vi "Open Playback Files Crop Utility.vi"(8 "error in (no error)":errorcluster, 11 "Frame Grabber Data In":T2={"Camera Session"="", "Frame"=refnum, "AVI Refnum"=refnum, "Codecs"=[], "Frame number"=0, "Tracking File Refnum"=refnum, "Tick Count"=0, "Probe Object"=refnum, "Playback Probe Data"=[], "Rigid Body"={"Position"={"x (mm)"=0.0, "y (mm)"=0.0, "z (mm)"=0.0}, "Orientation"={"Pitch (rad)"=0.0, "Yaw (rad)"=0.0, "Roll (rad)"=0.0}, "Quaternion"={"qx"=0.0, "qy"=0.0, "qz"=0.0, "qw"=0.0}, "Tracked?"=FALSE}, "Total no frames playback"=0, "Video FPS"=0.0, "Camera connected?"=FALSE, "Scene"=refnum, "Cropped Frame"=refnum, "Tracker FPS"=0.0, "Crop ROI"=[], "Presentation Values"=[], "Elapsed time (ms)"=0, "Camera frames playback"=0, "Refnums"={"Live Refnum"=refnum, "Record Refnum"=refnum, "Playback Refnum"=refnum, "Frame Slider Refnum"=refnum, "Pause Refnum"=refnum, "Home Refnum"=refnum, "Set Crop Refnum"=refnum, "Clear Crop Refnum"=refnum, "stop refnum"=refnum, "Playback Rate Refnum"=refnum, "Presentation Refnum"=refnum, "Crop Time Frame Slider Refnum"=refnum, "Cancel Save Refnum"=refnum, "Reverse Playback Refnum"=refnum, "Recording Settings Refnum"=refnum, "Continuous Playback Refnum"=refnum, "Annotation Refnum"=refnum, "Export All Refnum"=refnum, "Export List Refnum"=refnum, "Fill List Refnum"=refnum, "Save Crop Refnum"=refnum, "Skip Forward Refnum"=refnum, "Skip Backward Refnum"=refnum, "Single Annotation Refnum"=refnum, "Load Video Refnum"=refnum, "Set Start Refnum"=refnum, "Set End Refnum"=refnum, "Add to List Refnum"=refnum, "List of Annotations Refnum"=refnum, "Camera Frame Refnum"=refnum, "Load Image Refnum"=refnum, "Saving Refnum"=refnum}, "Dimensions"={"Probe Dimensions"={"Probe Width"=0.0, "Probe Depth"=1.0, "Probe Height"=0.0}, "Room Dimensions"={"Room Width"=0.0, "Room Depth"=0.0, "Room Height"=0.0}}, "Playback Data As Strings"=[], "Cropped Tracking File Refnum"=refnum, "Cropped AVI Refnum"=refnum, "Header"=[], "Total euclidian distance"=0.0, "Annotation File Path"=path "", "Playback File Path"=path "", "Size per frame"=0.0, "Ground Truth File Refnum"=refnum, "Annotation Array"=[], "Annotation TIFFs Folder"=path "", "overwriting open file?"=FALSE, "Image Sequence"=[], "Video/Image Flag"=enum."Playback Video Frame", "Image sequence?"=FALSE, "Image sequence filenames"=[], "Mask"=refnum}) -> (0 "error out":errorcluster, 1 "Playback Video":path, 2 "both exist and open?":bool, 3 "Frame Grabber Data Out":T2={"Camera Session"="", "Frame"=refnum, "AVI Refnum"=refnum, "Codecs"=[], "Frame number"=0, "Tracking File Refnum"=refnum, "Tick Count"=0, "Probe Object"=refnum, "Playback Probe Data"=[], "Rigid Body"={"Position"={"x (mm)"=0.0, "y (mm)"=0.0, "z (mm)"=0.0}, "Orientation"={"Pitch (rad)"=0.0, "Yaw (rad)"=0.0, "Roll (rad)"=0.0}, "Quaternion"={"qx"=0.0, "qy"=0.0, "qz"=0.0, "qw"=0.0}, "Tracked?"=FALSE}, "Total no frames playback"=0, "Video FPS"=0.0, "Camera connected?"=FALSE, "Scene"=refnum, "Cropped Frame"=refnum, "Tracker FPS"=0.0, "Crop ROI"=[], "Presentation Values"=[], "Elapsed time (ms)"=0, "Camera frames playback"=0, "Refnums"={"Live Refnum"=refnum, "Record Refnum"=refnum, "Playback Refnum"=refnum, "Frame Slider Refnum"=refnum, "Pause Refnum"=refnum, "Home Refnum"=refnum, "Set Crop Refnum"=refnum, "Clear Crop Refnum"=refnum, "stop refnum"=refnum, "Playback Rate Refnum"=refnum, "Presentation Refnum"=refnum, "Crop Time Frame Slider Refnum"=refnum, "Cancel Save Refnum"=refnum, "Reverse Playback Refnum"=refnum, "Recording Settings Refnum"=refnum, "Continuous Playback Refnum"=refnum, "Annotation Refnum"=refnum, "Export All Refnum"=refnum, "Export List Refnum"=refnum, "Fill List Refnum"=refnum, "Save Crop Refnum"=refnum, "Skip Forward Refnum"=refnum, "Skip Backward Refnum"=refnum, "Single Annotation Refnum"=refnum, "Load Video Refnum"=refnum, "Set Start Refnum"=refnum, "Set End Refnum"=refnum, "Add to List Refnum"=refnum, "List of Annotations Refnum"=refnum, "Camera Frame Refnum"=refnum, "Load Image Refnum"=refnum, "Saving Refnum"=refnum}, "Dimensions"={"Probe Dimensions"={"Probe Width"=0.0, "Probe Depth"=1.0, "Probe Height"=0.0}, "Room Dimensions"={"Room Width"=0.0, "Room Depth"=0.0, "Room Height"=0.0}}, "Playback Data As Strings"=[], "Cropped Tracking File Refnum"=refnum, "Cropped AVI Refnum"=refnum, "Header"=[], "Total euclidian distance"=0.0, "Annotation File Path"=path "", "Playback File Path"=path "", "Size per frame"=0.0, "Ground Truth File Refnum"=refnum, "Annotation Array"=[], "Annotation TIFFs Folder"=path "", "overwriting open file?"=FALSE, "Image Sequence"=[], "Video/Image Flag"=enum."Playback Video Frame", "Image sequence?"=FALSE, "Image sequence filenames"=[], "Mask"=refnum}, 4 "Annotation List":T1[](array[typedef]) {"Frame Start" min=0}, 5 "Number of Playback Frames":i32, 7 "Number of Camera Frames":u32)   [LabVIEW 2017]
uses:
  Controls/Frame Grabber Data.ctl
  <vilib>/userdefined/High Color/IMAQdx.ctl
  <vilib>/vision/Image Controls.llb/IMAQ Image.ctl
  <vilib>/vision/Avi.llb/IMAQ AVI2 Refnum.ctl
  Controls/Rigid Body Info.ctl
  Controls/Position.ctl
  Controls/Orientation.ctl
  Controls/Refnums.ctl
  Controls/Recording Settings.ctl
  Controls/Operator Settings.ctl
  Controls/Operator.ctl
  Controls/Patient Settings.ctl
  Controls/Dimensions.ctl
  Controls/Room Dimensions.ctl
  Controls/Crop Video State.ctl
  Controls/Annotation Sequence Details.ctl
  <vilib>/Utility/file.llb/Read Delimited Spreadsheet (string).vi
  <vilib>/vision/NI_Vision_Development_Module.lvlib
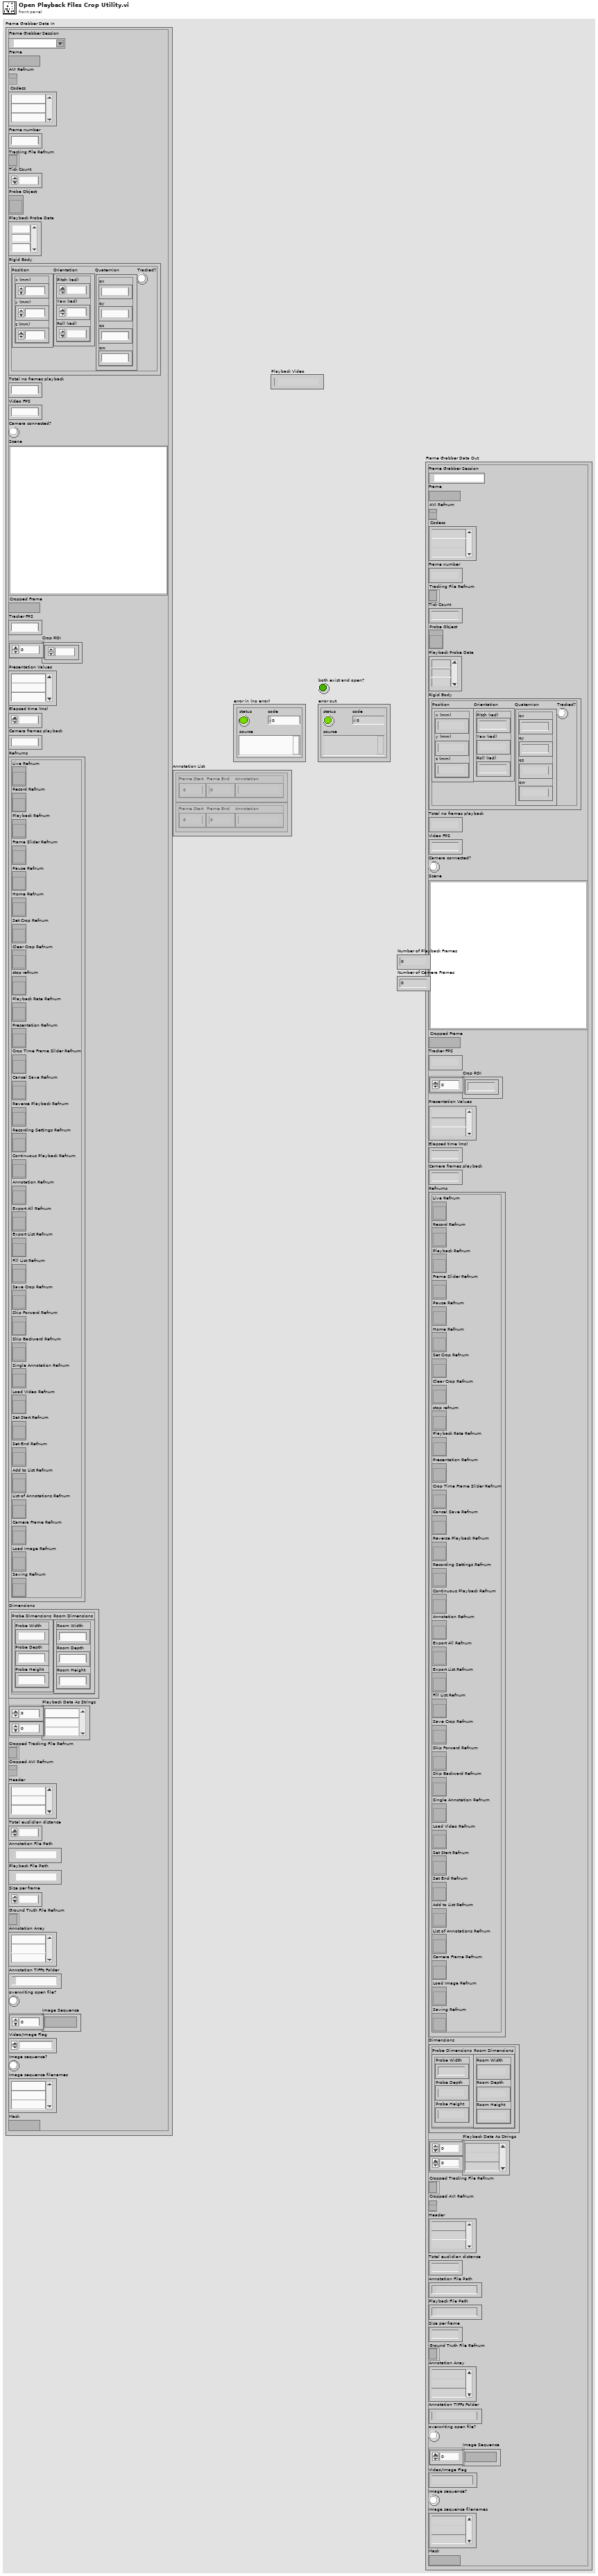
[diagram p1: front panel]
types:
  T1 = typedef "Annotation Sequence Details.ctl" = cluster{"Frame Start":i32, "Frame End":i32, "Annotation":string}
  T2 = typedef "Frame Grabber Data.ctl" = cluster{"Camera Session":T3, "Frame":T4, "AVI Refnum":T5, "Codecs":string[], "Frame number":u32, "Tracking File Refnum":refnum<file>, "Tick Count":u32, "Probe Object":refnum<vi>, "Playback Probe Data":dbl[][], "Rigid Body":T6, "Total no frames playback":i32, "Video FPS":dbl, "Camera connected?":bool, "Scene":refnum<vi>, "Cropped Frame":T4, "Tracker FPS":dbl, "Crop ROI":i32[], "Presentation Values":string[], "Elapsed time (ms)":u32, "Camera frames playback":u32, "Refnums":T9, "Dimensions":T10, "Playback Data As Strings":string[][], "Cropped Tracking File Refnum":refnum<file>, "Cropped AVI Refnum":T5, "Header":string[], "Total euclidian distance":dbl, "Annotation File Path":path, "Playback File Path":path, "Size per frame":dbl, "Ground Truth File Refnum":refnum<file>, "Annotation Array":string[], "Annotation TIFFs Folder":path, "overwriting open file?":bool, "Image Sequence":T4[], "Video/Image Flag":T12, "Image sequence?":bool, "Image sequence filenames":string[], "Mask":T4}
  T3 = typedef "IMAQdx.ctl" = refnum<k21>
  T4 = typedef "IMAQ Image.ctl" = refnum<image>
  T5 = typedef "IMAQ AVI2 Refnum.ctl" = refnum<k20>
  T6 = typedef "Rigid Body Info.ctl" = cluster{"Position":T7, "Orientation":T8, "Quaternion":cluster{"qx":sgl, "qy":sgl, "qz":sgl, "qw":sgl}, "Tracked?":bool}
  T7 = typedef "Position.ctl" = cluster{"x (mm)":sgl, "y (mm)":sgl, "z (mm)":sgl}
  T8 = typedef "Orientation.ctl" = cluster{"Pitch (rad)":sgl, "Yaw (rad)":sgl, "Roll (rad)":sgl}
  T9 = typedef "Refnums.ctl" = cluster{"Live Refnum":refnum<vi>, "Record Refnum":refnum<vi>, "Playback Refnum":refnum<vi>, "Frame Slider Refnum":refnum<vi>, "Pause Refnum":refnum<vi>, "Home Refnum":refnum<vi>, "Set Crop Refnum":refnum<vi>, "Clear Crop Refnum":refnum<vi>, "stop refnum":refnum<vi>, "Playback Rate Refnum":refnum<vi>, "Presentation Refnum":refnum<vi>, "Crop Time Frame Slider Refnum":refnum<vi>, "Cancel Save Refnum":refnum<vi>, "Reverse Playback Refnum":refnum<vi>, "Recording Settings Refnum":refnum<vi>, "Continuous Playback Refnum":refnum<vi>, "Annotation Refnum":refnum<vi>, "Export All Refnum":refnum<vi>, "Export List Refnum":refnum<vi>, "Fill List Refnum":refnum<vi>, "Save Crop Refnum":refnum<vi>, "Skip Forward Refnum":refnum<vi>, "Skip Backward Refnum":refnum<vi>, "Single Annotation Refnum":refnum<vi>, "Load Video Refnum":refnum<vi>, "Set Start Refnum":refnum<vi>, "Set End Refnum":refnum<vi>, "Add to List Refnum":refnum<vi>, "List of Annotations Refnum":refnum<vi>, "Camera Frame Refnum":refnum<vi>, "Load Image Refnum":refnum<vi>, "Saving Refnum":refnum<vi>}
  T10 = typedef "Dimensions.ctl" = cluster{"Probe Dimensions":cluster{"Probe Width":sgl, "Probe Depth":sgl, "Probe Height":sgl}, "Room Dimensions":T11}
  T11 = typedef "Room Dimensions.ctl" = cluster{"Room Width":dbl, "Room Depth":dbl, "Room Height":dbl}
  T12 = typedef "Crop Video State.ctl" = enum16{"Init", "Wait", "Load Image", "Load Video", "Play/Pause", "Playback Video Frame", "Display Image", "Save Image Sequence", "Save Video", "Export List", "Export All", "Close", "Set Crop Area", "Reset Crop Area", "Crop Inside", "Crop Outside", "Multi-Crop", "Re-Open Files", "Annotate Frame", "Annotate Clip", "Add to List", "Fill List", "Set Start", "Set End", "Error Handling", "Shutdown"}
  T13 = enum16{"open", "replace", "create", "open or create", "replace or create", "replace or create with confirmation"}
  T14 = typedef "IMAQ Rectangle" = cluster{"Left":i32, "Top":i32, "Right":i32, "Bottom":i32, "Rotation":dbl}
  T15 = enum8{"Enabled", "Disabled", "Disabled and Grayed Out"}
  T16 = cluster{"Width":u32, "Height":u32, "Frames Per Second":u32, "Codec":string, "Has Data":bool}
  T17 = cluster{"Scale.Range:Minimum":i32, "Number of Frames":u32, "Scale.Range:Minimum":i32}
  T18 = typedef "ROI Descriptor" = cluster{"Global Rectangle":i32[], "Contours":cluster{"ID":enum32{"External", "Internal"}, "Type":u32, "Coordinates":i32[]}[]}
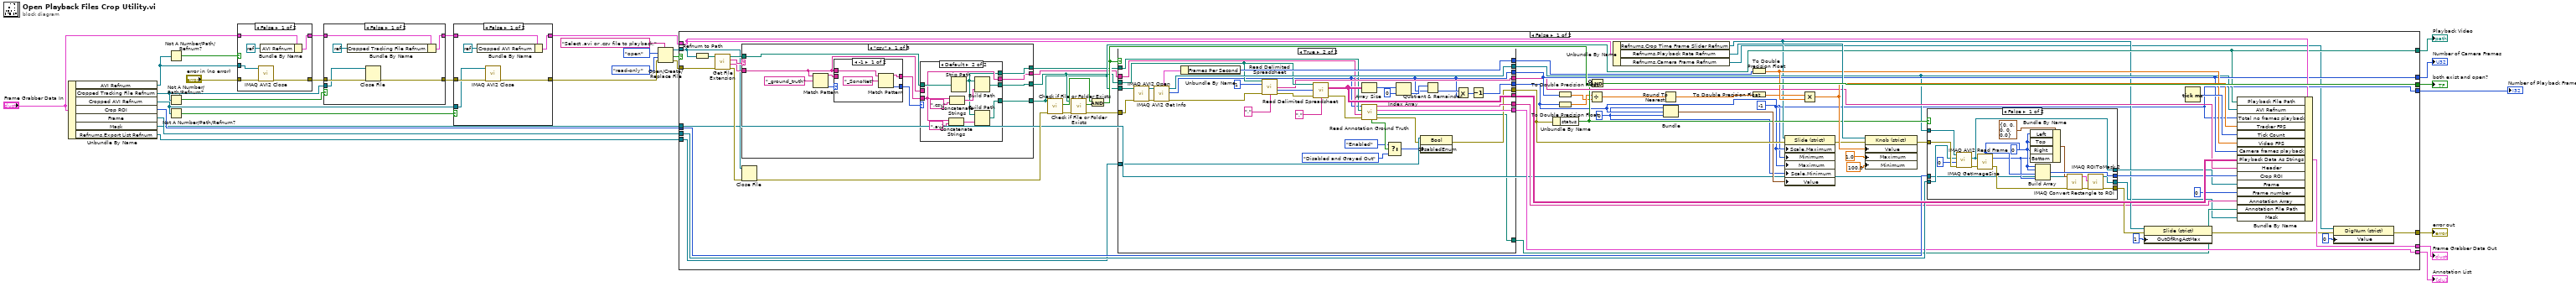
[diagram p0: block diagram]
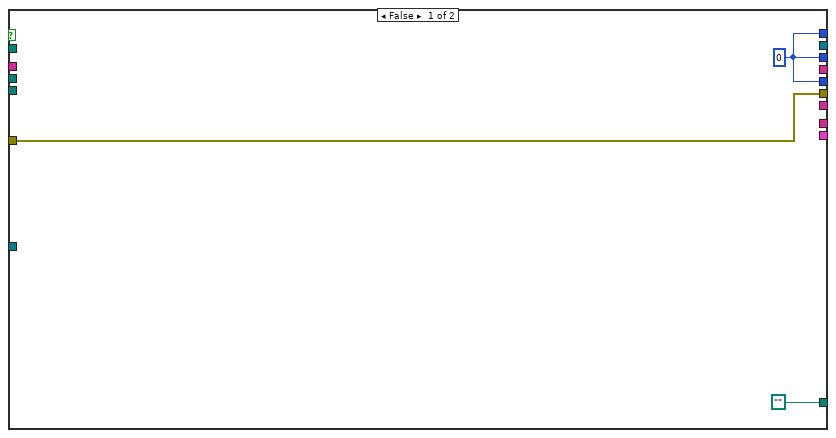
[diagram p6: hidden frame]
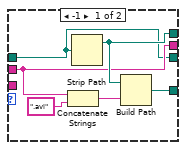
[diagram p8: hidden frame]
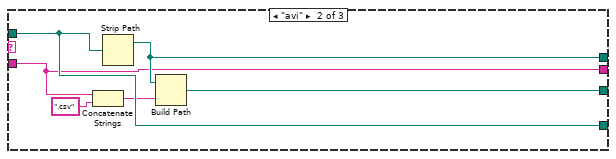
[diagram p9: hidden frame]
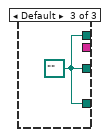
[diagram p10: hidden frame]
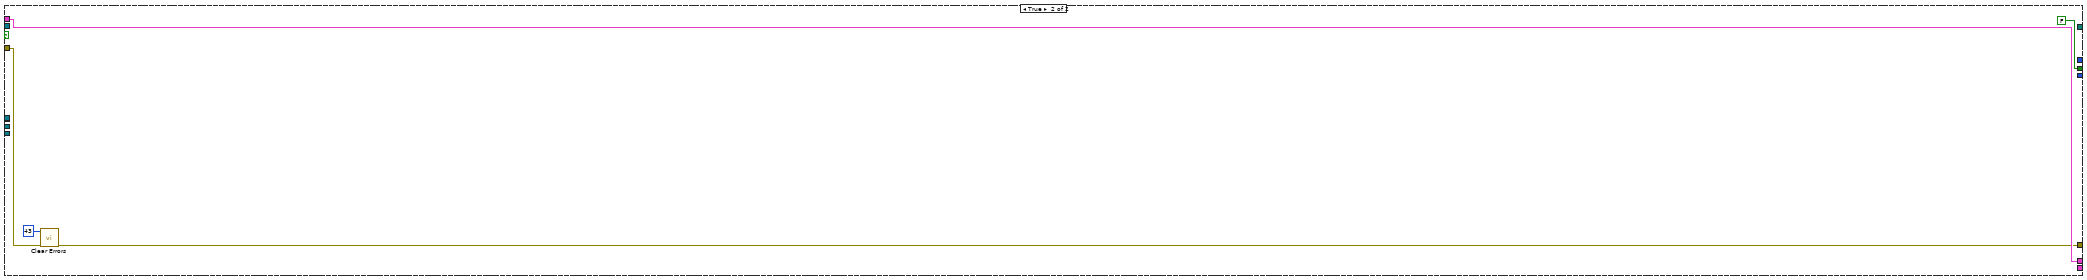
[diagram p11: hidden frame]
diagram:
  n1 = Unbundle By Name("Frame Grabber Data In") -> ("AVI Refnum"=w12:T5, "Cropped Tracking File Refnum"=w13:refnum<file>, "Cropped AVI Refnum"=w8:T5, "Crop ROI"=w5:i32[], "Frame"=w4:T4, "Mask"=w1:T4, "Refnums.Export List Refnum"=w2:refnum<vi>)
  n2 = Not A Number/Path/Refnum?(number/path/refnum=w12) -> (NaN/Path/Refnum?=w17:bool)
  n3 = Not A Number/Path/Refnum?(number/path/refnum=w13) -> (NaN/Path/Refnum?=w20:bool)
  n4 = Not A Number/Path/Refnum?(number/path/refnum=w8) -> (NaN/Path/Refnum?=w19:bool)
  n5 = case shown="False" w17 {
    tunnel: "error in (no error)" -> [w37 w39]
    tunnel: [w36 w39] -> w15
    tunnel: "Frame Grabber Data In" -> [w35 w38]
    tunnel: w12 -> [w34 _]
    tunnel: [w33 w38] -> w11
    frame False {
      n6 = call "IMAQ AVI2 Close"("error in (no error)"=w37, "AVI Refnum"=w34) -> ("error out"=w36:errorcluster)  [unwired: 9 in]
      n7 = Bundle By Name(cluster=w35, "AVI Refnum"=refnum<k0> refnum) -> (w33:T2)
    }
    frame True {
    }
  }
  n8 = case shown="False" w20 {
    tunnel: w15 -> [w45 w47]
    tunnel: [w44 w47] -> w21
    tunnel: w11 -> [w43 w46]
    tunnel: w13 -> [w42 _]
    tunnel: [w40 w46] -> w10
    frame False {
      n9 = Bundle By Name(cluster=w43, "Cropped Tracking File Refnum"=refnum<k0> refnum) -> (w40:T2)
      n10 = Close File(refnum=w42, error in=w45) -> (error out=w44:errorcluster)  [unwired: 1 out]
    }
    frame True {
    }
  }
  n11 = case shown="False" w19 {
    tunnel: w21 -> [w53 w55]
    tunnel: [w52 w55] -> w18
    tunnel: w10 -> [w51 w54]
    tunnel: [w50 w54] -> w9
    tunnel: w8 -> [w48 _]
    frame False {
      n12 = Bundle By Name(cluster=w51, "Cropped AVI Refnum"=refnum<k0> refnum) -> (w50:T2)
      n13 = call "IMAQ AVI2 Close"("error in (no error)"=w53, "AVI Refnum"=w48) -> ("error out"=w52:errorcluster)  [unwired: 9 in]
    }
    frame True {
    }
  }
  n14 = Open/Create/Replace File(error in=w18, prompt="Select .avi or .csv file to playback.", operation (0:open)=T13."open", access (0:read/write)=enum16{"read/write", "read-only", "write-only"}."read-only") -> (refnum out=w30:refnum<file>, cancelled=w24:bool, error out=w31:errorcluster)  [unwired: 2 in]
  n15 = case shown="False" w24 {
    tunnel: w31 -> [w117 w219]
    tunnel: w30 -> [w103 _]
    tunnel: w9 -> [w107 w221]
    tunnel: [w111 FALSE] -> w26
    tunnel: [w110 w221] -> w25
    tunnel: [w77 _] -> w23
    tunnel: [w70 w217] -> w22
    tunnel: [w72 _] -> w7
    tunnel: [w89 _] -> w6
    tunnel: w5 -> [w85 _]
    tunnel: w4 -> [w82 _]
    tunnel: [w66 _] -> w3
    tunnel: w2 -> [w60 _]
    tunnel: w1 -> [w56 _]
    frame False {
      w62 = 0 ("Scale.Range:Minimum")
      n16 = Refnum to Path(1:w103) -> (0:w116:path)
      n17 = call <vilib>:"Get File Extension.vi"("error in (no error)"=w117, "file"=w116) -> ("error out"=w104:errorcluster, "filename without extension"=w114:string, "lowercase file extension"=w115:string, "dup file"=w113:path)  [unwired: 5 in, 1 out]
      n18 = case shown="\"csv\"" w115 {
        tunnel: w114 -> [w181 w210 _]
        tunnel: w113 -> [w188 w214 _]
        tunnel: [w187 w214 w216] -> w77
        tunnel: [w183 w212 w216] -> w101
        tunnel: [w186 w211 w216] -> w64
        tunnel: [w184 w210 _] -> w63
        frame "csv" {
          n19 = Match Pattern(string=w181, regular expression="_ground_truth") -> (before substring=w179:string, offset past match=w182:i32)  [unwired: 1 in, 2 out]
          n20 = case shown="-1" w182 {
            selector: w182 -> [_ w194]
            tunnel: w181 -> [w191 _]
            tunnel: [w190 w194] -> w180
            tunnel: w179 -> [_ w193]
            tunnel: [w189 w193] -> w178
            frame -1 {
              n21 = Match Pattern(string=w191, regular expression="_SonoNet") -> (before substring=w189:string, offset past match=w190:i32)  [unwired: 1 in, 2 out]
            }
            frame Default {
            }
          }
          n22 = case shown="Default" w180 {
            tunnel: w188 -> [w195 w205]
            tunnel: [w198 w207] -> w187
            tunnel: [w197 w202] -> w186
            tunnel: w181 -> [w196 _]
            tunnel: w178 -> [_ w203]
            tunnel: [w196 w203] -> w184
            tunnel: [w195 w201] -> w183
            frame -1 {
              n23 = Concatenate Strings(w196, ".avi" ("string")) -> (w199:string)
              n24 = Strip Path(path=w195) -> (stripped path=w197:path)  [unwired: 1 out]
              n25 = Build Path(base path=w197, name or relative path=w199) -> (appended path=w198:path)
            }
            frame Default {
              n26 = Concatenate Strings(w203, ".avi" ("string")) -> (w208:string)
              n27 = Concatenate Strings(w203, ".csv" ("string")) -> (w204:string)
              n28 = Strip Path(path=w205) -> (stripped path=w202:path)  [unwired: 1 out]
              n29 = Build Path(base path=w202, name or relative path=w204) -> (appended path=w201:path)
              n30 = Build Path(base path=w202, name or relative path=w208) -> (appended path=w207:path)
            }
          }
        }
        frame "avi" {
          n31 = Concatenate Strings(w210, ".csv" ("string")) -> (w213:string)
          n32 = Strip Path(path=w214) -> (stripped path=w211:path)  [unwired: 1 out]
          n33 = Build Path(base path=w211, name or relative path=w213) -> (appended path=w212:path)
        }
        frame Default {
          w216 = path "" ("dup file")
        }
      }
      n34 = Close File(refnum=w103, error in=w104) -> (error out=w58:errorcluster)  [unwired: 1 out]
      n35 = call <vilib>:"Check if File or Folder Exists.vi"("error in (no error)"=w58, "path"=w77) -> ("error out"=w99:errorcluster, "file or folder exists?"=w102:bool)  [unwired: 7 in, 1 out]
      n36 = call <vilib>:"Check if File or Folder Exists.vi"("error in (no error)"=w99, "path"=w101) -> ("error out"=w67:errorcluster, "file or folder exists?"=w100:bool)  [unwired: 7 in, 1 out]
      n37 = And(x=w102, y=w100) -> (x .and. y?=w112:bool)
      n38 = case shown="True" w112 {
        tunnel: w67 -> [w141 w156]
        tunnel: w77 -> [_ w177]
        tunnel: [w141 w147] -> w108
        tunnel: [_ w174] -> w83
        tunnel: w101 -> [_ w169]
        tunnel: [w140 w152] -> w89
        tunnel: [w140 w172] -> w105
        tunnel: [w140 w150] -> w72
        tunnel: [_ w166] -> w90
        tunnel: [_ w162] -> w88
        tunnel: [_ w160] -> w66
        tunnel: [_ w159] -> w65
        tunnel: w64 -> [_ w158]
        tunnel: w63 -> [_ w157]
        tunnel: w60 -> [_ w149]
        tunnel: [path "" w142] -> w59
        frame False {
          w140 = 0 ("Number of Frames")
        }
        frame True {
          n39 = call "IMAQ AVI2 Open"("error in (no error)"=w156, "AVI File Path"=w177) -> ("error out"=w176:errorcluster, "AVI Refnum"=w175:T5)  [unwired: 8 in]
          n40 = call "IMAQ AVI2 Get Info"("error in (no error)"=w176, "AVI Refnum"=w175) -> ("error out"=w171:errorcluster, "Number of Frames"=w152:u32, "AVI Refnum (duplicate)"=w174:T5, "Frame Data"=w173:T16)  [unwired: 5 in, 1 out]
          n41 = Unbundle By Name(w173) -> ("Frames Per Second"=w172:u32)
          n42 = call-poly <vilib>:"Read Delimited Spreadsheet.vi"("file path (dialog if empty)"=w169, "number of rows (all:-1)"=1, "error in (no error)"=w171, "delimiter (\\t)"="," ("delimiter (\\t)")) -> ("first row"=w162:string[], "mark after read (chars.)"=w167:i32, "error out"=w168:errorcluster)  [unwired: 6 in, 3 out]
          n43 = call-poly <vilib>:"Read Delimited Spreadsheet.vi"("file path (dialog if empty)"=w169, "start of read offset (chars.:0)"=w167, "error in (no error)"=w168, "delimiter (\\t)"="," ("delimiter (\\t)")) -> ("all rows"=w166:string[][], "error out"=w155:errorcluster)  [unwired: 6 in, 4 out]
          n44 = Array Size(array=w166) -> (size(s)=w165:i32[])
          n45 = call "Read Annotation Ground Truth.vi"("Error In"=w155, "Filename without extension"=w157, "Folder"=w158, "Total no frames playback"=w152) -> ("Error Out"=w148:errorcluster, "annotation file path"=w142:path, "Annotation List"=w160:T1[], "Annotation array (strings)"=w159:string[], "annotation list exists?"=w146:bool)  [unwired: 3 in]
          n46 = Select(t=T15."Enabled" ("Disabled"), s=w146, f=T15."Disabled and Grayed Out") -> (s? t:f=w144:T15)
          n47 = Index Array(array=w165, index=0) -> (element=w154:i32)
          n48 = property class="Bool"(reference=w149, error in=w148, "DisabledEnum"=w144) -> (error out=w147:errorcluster)  [unwired: 1 out]
          n49 = Quotient & Remainder(x=w154, y=w152) -> (floor(x/y)=w153:u32)  [unwired: 1 out]
          n50 = Multiply(x=w153, y=w152) -> (x*y=w151:u32)
          n51 = Decrement(x=w151) -> (x-1=w150:u32)
        }
      }
      n52 = Unbundle By Name(w108) -> ("status"=w87:bool)
      n53 = To Double Precision Float(number=w89) -> (double precision float=w78:dbl)
      n54 = To Double Precision Float(number=w72) -> (double precision float=w79:dbl)
      n55 = Divide(x=w79, y=w78) -> (x/y=w106:dbl)
      n56 = Compound Arithmetic op=AND(invert w87, w112) -> (w111:bool)
      n57 = Unbundle By Name(w107) -> ("Refnums.Crop Time Frame Slider Refnum"=w74:refnum<vi>, "Refnums.Playback Rate Refnum"=w98:refnum<vi>, "Refnums.Camera Frame Refnum"=w69:refnum<vi>)
      n58 = Round To Nearest(number=w106) -> (nearest integer value=w80:dbl)
      n59 = Bundle("Scale.Range:Minimum"=w62, "Number of Frames"=w72, "Scale.Range:Minimum"=w62) -> (w91:T17)  [unwired: 1 in]
      n60 = To Double Precision Float(number=w105) -> (double precision float=w93:dbl)
      n61 = To Double Precision Float(number=w80) -> (double precision float=w92:dbl)
      n62 = property class="Slide (strict)"(reference=w74, error in=w108, "Scale.Maximum"=w72, "Minimum"=-1 ("Scale.Range:Minimum"), "Maximum"=w72, "Scale.Minimum"=w62, "Value"=w91) -> (error out=w96:errorcluster)  [unwired: 1 out]
      n63 = Multiply(x=w92, y=w93) -> (x*y=w97:dbl)
      n64 = property class="Knob (strict)"(reference=w98, error in=w96, "Value"=w97, "Maximum"=1.0 ("Data Entry Limits:Maximum"), "Minimum"=100.0 ("Data Entry Limits:Minimum")) -> (error out=w86:errorcluster)  [unwired: 1 out]
      n65 = case shown="False" w87 {
        tunnel: w86 -> [w135 w137]
        tunnel: w85 -> [_ w138]
        tunnel: [w133 w138] -> w84
        tunnel: w83 -> [w132 _]
        tunnel: w82 -> [w130 w136]
        tunnel: [w124 w137] -> w75
        tunnel: [w129 w136] -> w81
        tunnel: [w126 _] -> w57
        tunnel: w56 -> [w118 _]
        frame False {
          w122 = 0 ("element")
          n66 = call "IMAQ AVI2 Read Frame"("error in (no error)"=w135, "Frame Number"=u32 0, "Image"=w130, "AVI Refnum"=w132) -> ("error out"=w134:errorcluster, "Image Out"=w129:T4)  [unwired: 5 in, 1 out]
          n67 = call "IMAQ GetImageSize"("Image"=w129, "error in (no error)"=w134) -> ("Y Resolution"=w120:i32, "X Resolution"=w121:i32, "error out"=w125:errorcluster)  [unwired: 2 in]
          n68 = Bundle By Name(cluster=T14 {"Left"=0, "Top"=0, "Right"=0, "Bottom"=0, "Rotation"=0.0} ("Rectangle"), "Left"=w122, "Top"=w122, "Right"=w121, "Bottom"=w120) -> (w119:T14)
          n69 = Build Array(w122, w122, w121, w120) -> (w133:i32[])
          n70 = call "IMAQ Convert Rectangle to ROI"("error in (no error)"=w125, "Rectangle"=w119) -> ("error out"=w128:errorcluster, "ROI Descriptor"=w127:T18)  [unwired: 7 in]
          n71 = call "IMAQ ROIToMask 2"("error in (no error)"=w128, "ROI Descriptor"=w127, "Image"=w118) -> ("error out"=w124:errorcluster, "Image Out"=w126:T4)  [unwired: 6 in, 1 out]
        }
        frame True {
        }
      }
      n72 = property class="Slide (strict)"(reference=w74, error in=w75, "OutOfRngActMax"=u8 1 ("Response to Value Outside Limits:Maximum")) -> (error out=w71:errorcluster)  [unwired: 1 out]
      n73 = Tick Count (ms)() -> (millisecond timer value=w109:u32)
      n74 = Bundle By Name(cluster=w107, "Playback File Path"=w77, "AVI Refnum"=w83, "Total no frames playback"=w72, "Tracker FPS"=w97, "Tick Count"=w109, "Video FPS"=w93, "Camera frames playback"=w89, "Playback Data As Strings"=w90, "Header"=w88, "Crop ROI"=w84, "Frame"=w81, "Frame number"=u32 0, "Annotation Array"=w65, "Annotation File Path"=w59, "Mask"=w57) -> (w110:T2)
      n75 = property class="DigNum (strict)"(reference=w69, error in=w71, "Value"=u32 0) -> (error out=w70:errorcluster)  [unwired: 1 out]
    }
    frame True {
      n76 = call <vilib>:"Clear Errors.vi"("error in (no error)"=w219, "specific error code to clear (0: all)"=43) -> ("error out"=w217:errorcluster)  [unwired: 4 in, 1 out]
    }
  }
  "both exist and open?" <- w26
  "Frame Grabber Data Out" <- w25
  "Playback Video" <- w23
  "error out" <- w22
  "Number of Playback Frames" <- w7
  "Number of Camera Frames" <- w6
  "Annotation List" <- w3
